vi "Configure Digital Channel.vi"(7 "Enable Digital Channel (T: Enable)":bool=TRUE, 8 "error in (no error)":errorcluster, 9 "Threshold (1.4 V)":dbl=1.4, 10 "Digital Channel (14: Digital Channel 0)":u16(ring)=14 items=["Digital Channel 0"=14, "Digital Channel 1"=15, "Digital Channel 2"=16, "Digital Channel 3"=17, "Digital Channel 4"=18, "Digital Channel 5"=19, "Digital Channel 6"=20, "Digital Channel 7"=21, "Digital Channel 8"=22, "Digital Channel 9"=23, "Digital Channel 10"=24, "Digital Channel 11"=25, "Digital Channel 12"=26, "Digital Channel 13"=27, "Digital Channel 14"=28, "Digital Channel 15"=29], 11 "VISA resource name":refnum<visa-resource-name>) -> (0 "error out":errorcluster, 3 "VISA resource name out":refnum<visa-resource-name>)   [LabVIEW 2010, in "Tektronix DPO MSO 2000 4000 Series.lvlib"]
doc: "Enables, disables and configures the digital channel settings of the MSO model oscilloscopes. \n\n<B>Note:</B>\n This VI only applies to MSO and MDO models and not DPO models."
uses:
  <instrlib>/Tektronix DPO MSO 2000 4000 Series/Tektronix DPO MSO 2000 4000 Series.lvlib
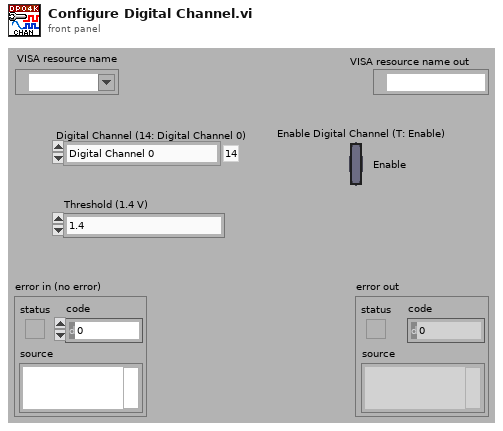
[diagram p1: front panel]
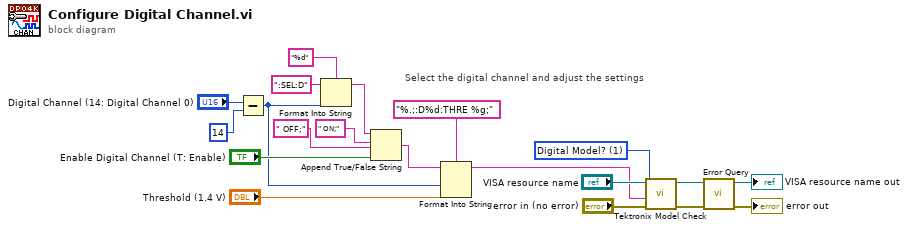
[diagram p0: block diagram]
diagram:
  w1 = u16 1 items=["Two-channel?", "Digital Model?", "Four-channel?", "RF Model?"] ("Oscilloscope Model Tests (3: RF Model?)")
  # "Select the digital channel and adjust the settings"
  n1 = Subtract(x="Digital Channel (14: Digital Channel 0)", y=u16 14) -> (x-y=w7:u16)
  n2 = Format Into String(format string="%d", initial string=":SEL:D", w7) -> (resulting string=w17:string)  [unwired: 1 in, 1 out]
  n3 = Append True/False String(1:"Enable Digital Channel (T: Enable)", 2:" OFF;" ("false string"), 3:" ON;" ("true string"), 4:w17) -> (0:w14:string)
  n4 = Format Into String(format string="%.;:D%d:THRE %g;" ("initial string"), initial string=w14, w7, "Threshold (1.4 V)") -> (resulting string=w2:string)  [unwired: 1 in, 1 out]
  n5 = call <instrlib>:"Tektronix Model Check.vi"("error in (no error)"="error in (no error)", "Command String"=w2, "Oscilloscope Model Tests (3: RF Model?)"=w1, "VISA resource name"="VISA resource name") -> ("error out"=w4:errorcluster, "VISA resource name out"=w3:refnum<visa-resource-name>)  [unwired: 6 in]
  n6 = call <instrlib>:"Error Query.vi"("error in (no error)"=w4, "VISA resource name"=w3) -> ("error out"=→"error out":errorcluster, "VISA resource name out"=→"VISA resource name out":refnum<visa-resource-name>)  [unwired: 6 in, 2 out]
